vi "XML - Get absolute RT Driver VI path for TARGET.vi"(7 "Target Type (Windows)":T1, 10 "CD Template":refnum<class "NIVS_CD Template.lvclass">, 11 "Project Name":string) -> (3 "Relative RT Driver TARGET path":path)   [LabVIEW 2017, in "NIVS_Consolidated_CDW_MetaDataObj.lvclass"]
doc: "Create the absolute path for the RT Driver VI inside the Configuration LLB for the <B>RT Target</B> based on the name and execution mode of the new custom device."
uses:
  NIVS_Consolidated_CDW_MetaDataObj.lvclass
  Target Type.ctl
  Template Classes/NIVS_CD Template/NIVS_CD Template.lvclass
  CD Engine lvlib.ctl
  Build Spec Engine.ctl
  Build Spec Engine.vi
  CD Engine lvlib.vi
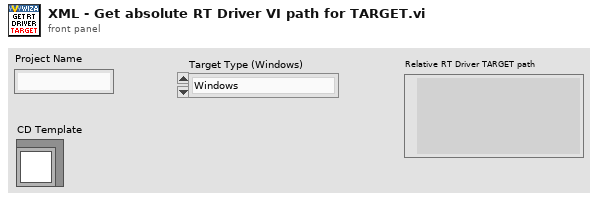
[diagram p1: front panel]
types:
  T1 = typedef "NIVS_Consolidated_CDW_MetaDataObj.lvclass/Target Type.ctl" = enum16{"Windows", "VxWorks", "Pharlap", "Linux 32 ARM", "Linux x64"}
  T2 = typedef "NIVS_Consolidated_CDW_MetaDataObj.lvclass/CD Engine lvlib.ctl" = enum16{"LibraryFileName", "LibraryFolderName", "Engine.FolderName", "Engine.Init.FolderName", "Engine.Run.FolderName", "Engine.Shutdown.FolderName", "Types.FolderName", "Engine.RT Driver VI.TemplatePath", "Engine.RT Driver VI.FileName", "Engine.RTStateVariables.Name", "Engine.RTStateVariables.Name.NoExtension", "Engine.Async.NameExtension", "Engine.Async.TemplateName"}
  T3 = typedef "NIVS_Consolidated_CDW_MetaDataObj.lvclass/Build Spec Engine.ctl" = enum16{"Destinations.LLBWindowsFileName", "Destinations.LLBVxWorksFileName", "Destinations.LLBPharlapFileName", "Destinations.LLBLinuxARMFileName", "Destinations.LLBLinux64FileName"}
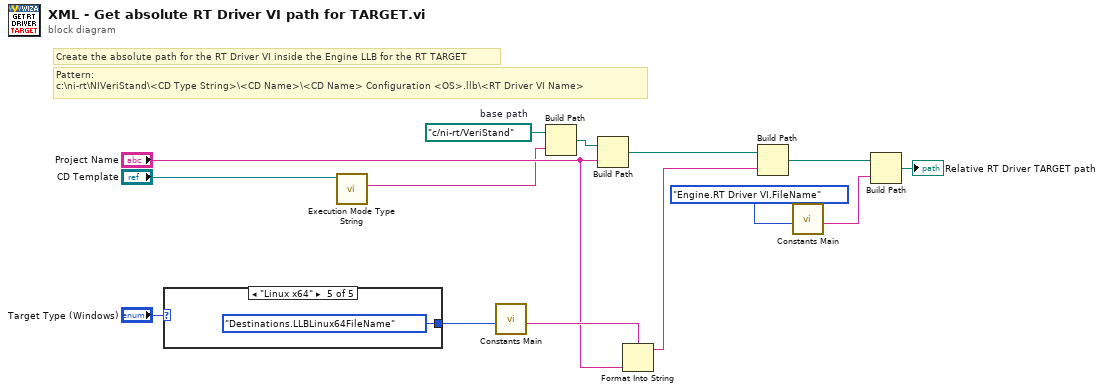
[diagram p0: block diagram]
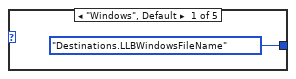
[diagram p2: hidden frame]
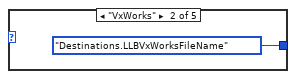
[diagram p3: hidden frame]
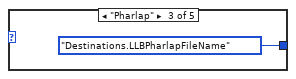
[diagram p4: hidden frame]
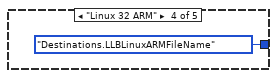
[diagram p5: hidden frame]
diagram:
  w8 = path "c:/ni-rt/VeriStand"  # base path
  # "Create the absolute path for the RT Driver VI inside the Engine LLB for the RT TARGET"
  # "Pattern:\nc:\\ni-rt\\NIVeriStand\\<CD Type String>\\<CD Name>\\<CD Name> Configuration <OS>.llb\\<RT Driver VI Name>"
  n1 = case shown="\"Linux x64\"" "Target Type (Windows)" {
    tunnel: [Build_Spec_Engine."Destinations.LLBWindowsFileName" ("Action") Build_Spec_Engine."Destinations.LLBVxWorksFileName" ("Action") Build_Spec_Engine."Destinations.LLBPharlapFileName" ("Action") Build_Spec_Engine."Destinations.LLBLinuxARMFileName" ("Action") Build_Spec_Engine."Destinations.LLBLinux64FileName" ("Action")] -> w9
    frame "Windows", Default {
    }
    frame "VxWorks" {
    }
    frame "Pharlap" {
    }
    frame "Linux 32 ARM" {
    }
    frame "Linux x64" {
    }
  }
  n2 = call-dynamic "Execution Mode Type String.vi"("CD Template"="CD Template") -> ("Execution Mode Type String"=w1:string)  [unwired: 10 in]
  n3 = call-poly "Constants Main.vi"("Action"=w9) -> ("Output"=w11:string)  [unwired: 10 in]
  n4 = Build Path(base path=w8, name or relative path=w1) -> (appended path=w7:path)
  n5 = Build Path(base path=w7, name or relative path="Project Name") -> (appended path=w10:path)
  n6 = Format Into String(format string=w11, "Project Name") -> (resulting string=w12:string)  [unwired: 2 in, 1 out]
  n7 = Build Path(base path=w10, name or relative path=w12) -> (appended path=w5:path)
  n8 = call-poly "Constants Main.vi"("Action"=CD_Engine_lvlib."Engine.RT Driver VI.FileName") -> ("Output"=w4:string)  [unwired: 10 in]
  n9 = Build Path(base path=w5, name or relative path=w4) -> (appended path=→"Relative RT Driver TARGET path":path)
